vi "subVi_extr_dias.vi"(1 "dias_edif 2":bool[](array[boolean])) -> (0 "dias 2":string)   [LabVIEW 2017]
panel:
  # "Lunes"
  # "Martes"
  # "Miercoles"
  # "Jueves"
  # "Viernes"
  # "Sabado"
  # "Domingo"
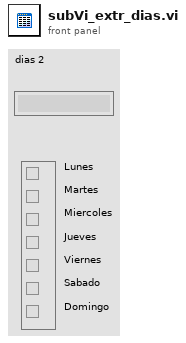
[diagram p1: front panel]
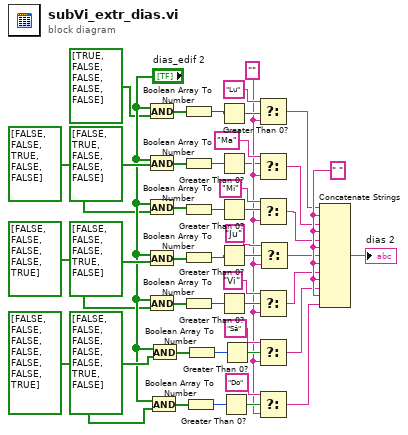
[diagram p0: block diagram]
diagram:
  w2 = ""
  w43 = " "
  n1 = And(x="dias_edif 2", y=bool[] [TRUE, FALSE, FALSE, FALSE, FALSE]) -> (x .and. y?=w33:bool[])
  n2 = And(x="dias_edif 2", y=bool[] [FALSE, TRUE, FALSE, FALSE, FALSE]) -> (x .and. y?=w32:bool[])
  n3 = And(x="dias_edif 2", y=bool[] [FALSE, FALSE, TRUE, FALSE, FALSE]) -> (x .and. y?=w31:bool[])
  n4 = And(x="dias_edif 2", y=bool[] [FALSE, FALSE, FALSE, TRUE, FALSE]) -> (x .and. y?=w30:bool[])
  n5 = And(x="dias_edif 2", y=bool[] [FALSE, FALSE, FALSE, FALSE, TRUE]) -> (x .and. y?=w29:bool[])
  n6 = And(x="dias_edif 2", y=bool[] [FALSE, FALSE, FALSE, FALSE, FALSE, FALSE, TRUE]) -> (x .and. y?=w40:bool[])
  n7 = And(x="dias_edif 2", y=bool[] [FALSE, FALSE, FALSE, FALSE, FALSE, TRUE, FALSE]) -> (x .and. y?=w37:bool[])
  n8 = Boolean Array To Number(Boolean array=w33) -> (number=w28:u32)
  n9 = Boolean Array To Number(Boolean array=w32) -> (number=w27:u32)
  n10 = Boolean Array To Number(Boolean array=w31) -> (number=w26:u32)
  n11 = Boolean Array To Number(Boolean array=w30) -> (number=w25:u32)
  n12 = Boolean Array To Number(Boolean array=w29) -> (number=w24:u32)
  n13 = Boolean Array To Number(Boolean array=w40) -> (number=w39:u32)
  n14 = Boolean Array To Number(Boolean array=w37) -> (number=w38:u32)
  n15 = Greater Than 0?(x=w28) -> (x > 0?=w22:bool)
  n16 = Greater Than 0?(x=w27) -> (x > 0?=w1:bool)
  n17 = Greater Than 0?(x=w26) -> (x > 0?=w18:bool)
  n18 = Greater Than 0?(x=w25) -> (x > 0?=w17:bool)
  n19 = Greater Than 0?(x=w24) -> (x > 0?=w19:bool)
  n20 = Greater Than 0?(x=w39) -> (x > 0?=w16:bool)
  n21 = Greater Than 0?(x=w38) -> (x > 0?=w15:bool)
  n22 = Select(t="Lu", s=w22, f=w2) -> (s? t:f=w21:string)
  n23 = Select(t="Ma", s=w1, f=w2) -> (s? t:f=w8:string)
  n24 = Select(t="Mi", s=w18, f=w2) -> (s? t:f=w7:string)
  n25 = Select(t="Vi", s=w19, f=w2) -> (s? t:f=w5:string)
  n26 = Select(t="Sá", s=w15, f=w2) -> (s? t:f=w4:string)
  n27 = Select(t="Do", s=w16, f=w2) -> (s? t:f=w3:string)
  n28 = Select(t="Ju", s=w17, f=w2) -> (s? t:f=w6:string)
  n29 = Concatenate Strings(w21, w43, w8, w43, w7, w43, w6, w43, w5, w43, w4, w43, w3) -> (→"dias 2":string)
